vi "Size to Smallest.vi"(9 "Secondary Array In":variant[](array[variant]), 11 "Primary Array In":variant[](array[variant])) -> (1 "Secondary Array Out":variant[](array[variant]), 3 "Primary Array Out":variant[](array[variant]))   [LabVIEW 2015]
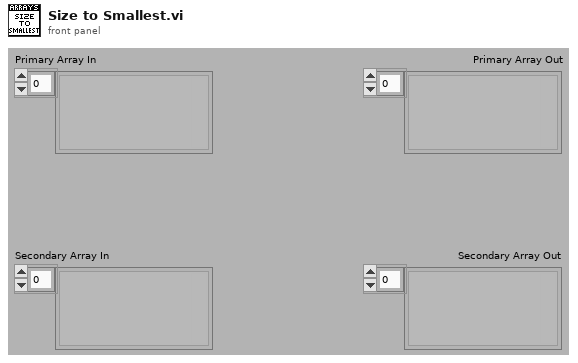
[diagram p1: front panel]
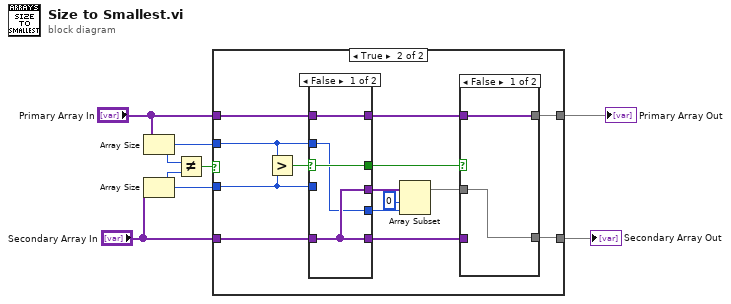
[diagram p0: block diagram]
diagram:
  n1 = Array Size(array="Primary Array In") -> (size(s)=w2:i32)
  n2 = Array Size(array="Secondary Array In") -> (size(s)=w1:i32)
  n3 = Not Equal?(x=w2, y=w1) -> (x != y?=w7:bool)
  n4 = case shown="True" w7 {
    tunnel: "Secondary Array In" -> [w9 w23]
    tunnel: [w9 w21] -> w5
    tunnel: "Primary Array In" -> [w8 w22]
    tunnel: [w8 w20] -> w3
    tunnel: w2 -> [_ w19]
    tunnel: w1 -> [_ w18]
    frame False {
    }
    frame True {
      n5 = Greater?(x=w19, y=w18) -> (0:w10:bool)
      n6 = case shown="False" w10 {
        selector: w10 -> [w29 w33]
        tunnel: [w30 w34] -> w14
        tunnel: w22 -> [w31 w34]
        tunnel: [w30 w35] -> w17
        tunnel: w23 -> [w30 w35]
        tunnel: [w31 w34] -> w16
        tunnel: [w29 w33] -> w15
        tunnel: w18 -> [_ w32]
        tunnel: [w28 w32] -> w12
        tunnel: w19 -> [w28 _]
        frame False {
        }
        frame True {
        }
      }
      n7 = Array Subset(array=w14, index=0, length=w12) -> (w13:variant[])
      n8 = case shown="False" w15 {
        tunnel: w13 -> [w25 w27]
        tunnel: [w25 w26] -> w21
        tunnel: w17 -> [_ w26]
        tunnel: w16 -> [w24 _]
        tunnel: [w24 w27] -> w20
        frame False {
        }
        frame True {
        }
      }
    }
  }
  "Secondary Array Out" <- w5
  "Primary Array Out" <- w3
